vi "Write topicName.vi"(10 "topicName":string, 11 "Topic in":refnum<class "Topic.lvclass">) -> (3 "Topic out":refnum<class "Topic.lvclass">)   [LabVIEW 2016, in "Topic.lvclass"]
uses:
  Topic.lvclass
  Topic.lvclass/Topic.ctl
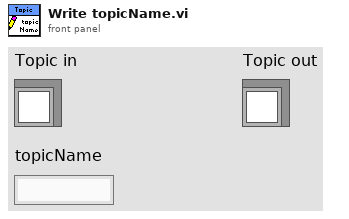
[diagram p1: front panel]
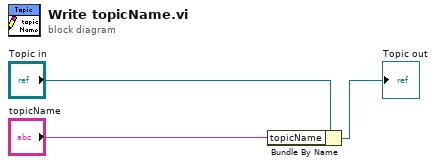
[diagram p0: block diagram]
diagram:
  n1 = Bundle By Name(cluster="Topic in", "topicName"="topicName") -> (→"Topic out":refnum<class "Topic.lvclass">)
